vi "LKIF_GetLight.vi"(8 "error in (no error)":errorcluster {"code" format="%x"}, 10 "PeakNo (0)":i32, 11 "HeadNo (0: Head A)":i32) -> (0 "error out":errorcluster {"code" format="%x"}, 1 "NumReaded":i32, 2 "Value":u8[](array[numeric]), 3 "MeasurePosition":i32[](array[numeric]))   [LabVIEW 2024, in "Keyence LK-G3000.lvlib"]
uses:
  Keyence LK-G3000.lvlib
  LkIF.dll
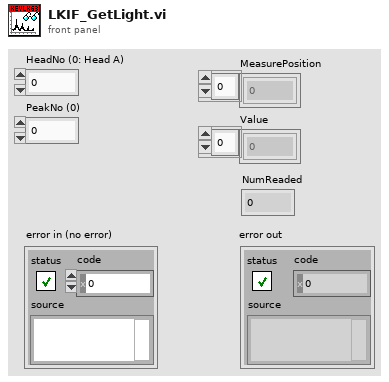
[diagram p1: front panel]
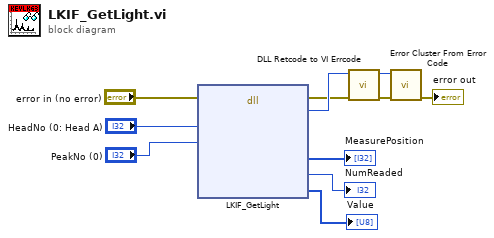
[diagram p0: block diagram]
diagram:
  n1 = dll-call lib="C:/Users/ff107/OneDrive/Documents/GitHub/PWC-OLS/Hardware Interface/Keyance Demo Code/Keyence LK-G3000/LkIF.dll" fn="LKIF_GetLight"(error in="error in (no error)", "HeadNo"="HeadNo (0: Head A)", "PeakNo"="PeakNo (0)") -> (error out=w2:errorcluster, "RC"=w3:i32, "MeasurePosition"=→"MeasurePosition":i32[], "NumReaded"=→"NumReaded":i32, "Value"=→"Value":u8[])  [unwired: 7 in, 1 out]
  n2 = call "DLL Retcode to VI Errcode.vi"("error in (no error)"=w2, "DLL Retcode"=w3) -> ("error out"=w11:errorcluster, "VI Errcode"=w10:i32)  [unwired: 8 in]
  n3 = call <vilib>:"Error Cluster From Error Code.vi"("error in (no error)"=w11, "error code (0)"=w10) -> ("error out"=→"error out":errorcluster)  [unwired: 7 in]
